vi "Subvi_Online_For_Offline_SWLDA_통합버전.vi"(0 "rate":dbl=500.0 caption="Rate" format="%0.2f", 1 "samples per channel":i32=25, 5 "Brain_data_source":dbl[][](array[numeric]) caption="EEG_Raw_Data" format="%0.3f", 7 "Target_Flash_Order":i64[][](array[numeric]), 8 "Value":T1, 9 "사용할 Parameter 갯수":i32=2, 10 "Weight":dbl[](array[numeric]), 11 "Path":path, 14 "Number":string, 16 "Matrix":T1, 17 "Channel selection":bool[](array[boolean])) -> (13 "LDA_Parameter":dbl[][](array[numeric]), 15 "EPR_발생_total":i16[](array[numeric]), 20 "output-0~8":i32, 22 "ERP_Parameters":dbl[][](array[numeric]))   [LabVIEW 2014]
uses:
  <vilib>/Analysis/Matrix/Datatypes/RealMatrix.ctl
  <vilib>/Analysis/3filter.llb/Filter Passband Type.ctl
  <vilib>/Analysis/baseanly.llb/Real A x B.vi
  <vilib>/Analysis/baseanly.llb/Mean (DBL).vi
  <vilib>/Analysis/3filter.llb/Butterworth Filter (DBL).vi
  <vilib>/Analysis/Matrix/Numeric/Conversions/Array To Matrix - RA.vi
  <vilib>/Analysis/Matrix/Numeric/Conversions/Array To Matrix - RA2.vi
  <vilib>/Analysis/Matrix/Numeric/Conversions/Matrix To Array - RM.vi
  <vilib>/Analysis/Matrix/Numeric/Multiply/Multiply - RM,RM.vi
  <vilib>/Analysis/Matrix/Numeric/Subtract/Subtract - RM,RM.vi
  <vilib>/Analysis/NI_AALBase.lvlib
  <vilib>/Analysis/Matrix/NI_Matrix.lvlib
  <vilib>/Utility/file.llb/Read From Spreadsheet File (DBL).vi
panel:
  out "Array 3":dbl[][](array[numeric])
  out "size(s)":i32[](array[numeric])
  out "A - B":T1
  out "Array 2":dbl[][](array[numeric])
  out "subarray":dbl[](array[numeric])
  out "Array":dbl[][](array[numeric])
  out "deleted portion":dbl[][](array[numeric])
  in  "LDA":path=path "C:/Users/Administrator/Desktop/공공복지안전사업연구-노수진/파일럿20130902/LDA_Matrix_Value.xls"
  out "#channel":i32
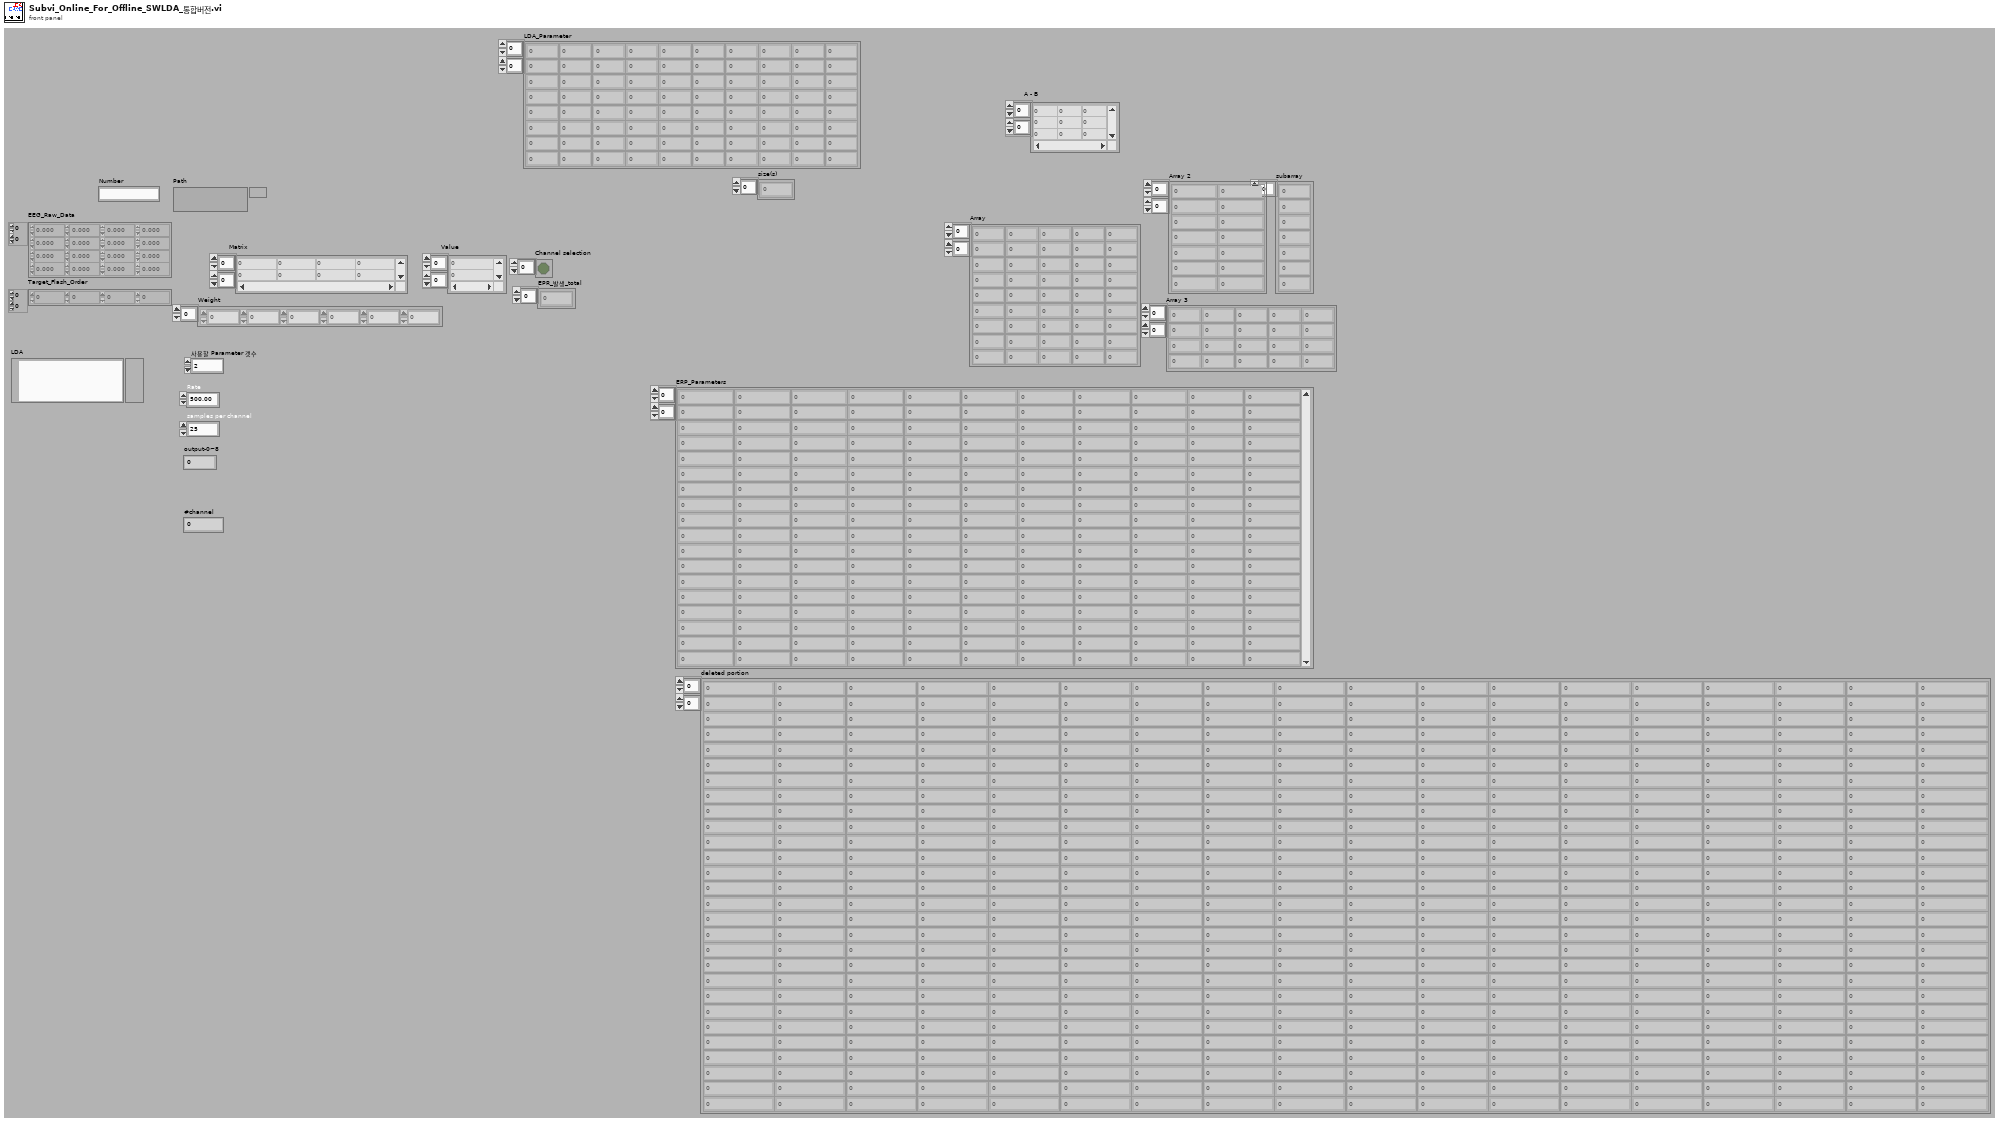
[diagram p1: front panel]
types:
  T1 = typedef "NI_Matrix.lvlib/RealMatrix.ctl" = dbl[][]
  T2 = typedef "NI_AALBase.lvlib/Filter Passband Type.ctl" = enum32{"Lowpass", "Highpass", "Bandpass", "Bandstop"}
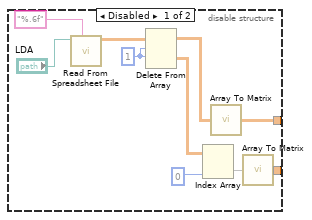
[diagram p3: hidden frame]
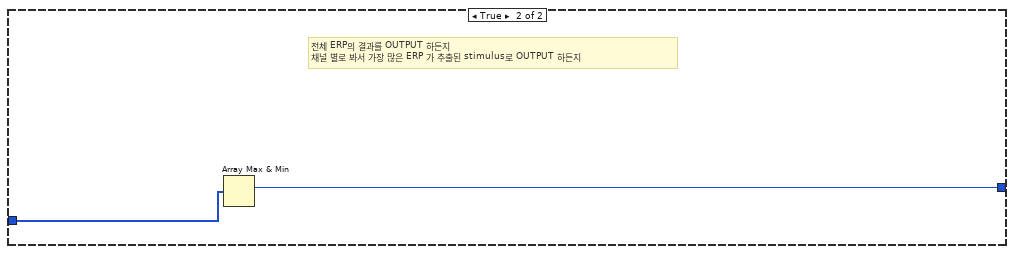
[diagram p4: hidden frame]
diagram:
  n1 = flat-sequence {
    tunnel: [w24] -> w19
    tunnel: [w48] -> w18
    tunnel: ["Target_Flash_Order"] -> w17
    tunnel: w19 -> [w48]
    tunnel: [w45] -> w16
    tunnel: w18 -> [w56]
    tunnel: w17 -> [w55]
    tunnel: w16 -> [w54]
    tunnel: [w52] -> w15
    tunnel: ["Weight"] -> w8
    tunnel: w15 -> [w183]
    tunnel: [w185] -> w14
    tunnel: [w185] -> w13
    tunnel: [w185] -> w12
    tunnel: w8 -> [w180]
    tunnel: [w180] -> w7
    tunnel: [w178] -> w5
    tunnel: w14 -> [_]
    tunnel: w13 -> [_]
    tunnel: w12 -> [w216]
    tunnel: [w219] -> w11
    tunnel: w7 -> [w218]
    tunnel: [w218] -> w6
    tunnel: w5 -> [w217]
    tunnel: [w216] -> w4
    tunnel: [w214] -> w2
    tunnel: w11 -> [w224]
    tunnel: [w224] -> w10
    tunnel: w6 -> [_]
    tunnel: w4 -> [w223]
    tunnel: [w223] -> w3
    tunnel: w2 -> [w222]
    tunnel: [w222] -> w1
    tunnel: [w227] -> w9
    tunnel: w10 -> [w228]
    tunnel: w3 -> [w226]
    tunnel: w1 -> [w225]
    tunnel: w9 -> [w233]
    frame #0 {
      n2 = Array Size(array="Brain_data_source") -> (size(s)=w25:i32[])
      n3 = Index Array(array=w25, index=1) -> (element=w27:i32)
      "#channel" <- w27
      n4 = for {
        N: w27 -> [_]
        tunnel: "Brain_data_source" -> [w32]
        shift-right: [w29] -> w21
        shift-left: dbl[][] [] ("Filtered X") -> [w30]
        tunnel: "Channel selection" -> [w28] mode=indexing
        i -> [w31]
        n5 = case shown="True" w28 {
          tunnel: w32 -> [_ w43]
          tunnel: w31 -> [_ w42]
          tunnel: w30 -> [w33 w36]
          tunnel: [w33 w35] -> w29
          frame False {
          }
          frame True {
            n6 = local read "rate"() -> (w37:dbl)
            n7 = Index Array(array=w43, index (col)=w42) -> (element=w41:dbl[])  [unwired: 1 in]
            n8 = call-poly <vilib>:"Butterworth Filter.vi"("filter type"=Filter_Passband_Type."Bandpass", "low cutoff freq: fl"=0.5, "high cutoff freq: fh"=30.0, "sampling freq: fs"=w37, "X"=w41) -> ("Filtered X"=w34:dbl[])  [unwired: 3 in, 1 out]
            n9 = Build Array (concatenate)(w36, w34) -> (w35:dbl[][])
          }
        }
      }
      n10 = Transpose 2D Array(2D array=w21) -> (transposed array=w24:dbl[][])
    }
    frame #1 {
      # "Bandpass per channel"
      # "20*9"
      n11 = Array Size(array="Target_Flash_Order") -> (size(s)=w47:i32[])
      n12 = Index Array(array=w47, index=1 ("인덱스")) -> (element=w45:i32)
    }
    frame #2 {
      (unwired) dbl[][] []
      (unwired) dbl[][] []
      n13 = for {
        N: w54 -> [_]
        tunnel: w56 -> [w69]
        tunnel: w55 -> [w68]
        shift-right: [w66] -> w52
        shift-left: dbl[][] [] -> [w65]
        shift-right: [w60] -> w50
        shift-left: dbl[][] [] -> [w59]
        tunnel: "Weight" -> [w58]
        i -> [w64]
        n14 = Index Array(array=w68, index (col)=w64) -> (element=w67:i64[])  [unwired: 1 in]
        n15 = flat-sequence {
          tunnel: w69 -> [w75]
          tunnel: w67 -> [w74]
          tunnel: [w73] -> w70
          tunnel: ["Path"] -> w63
          tunnel: ["Number"] -> w62
          tunnel: w70 -> [w136]
          tunnel: [w123] -> w57
          tunnel: w63 -> [_]
          tunnel: w62 -> [_]
          tunnel: [w118] -> w61
          tunnel: w58 -> [w126]
          frame #0 {
            # "10*600"
            # "Channel number"
            n16 = local read "samples per channel"() -> (w82:i32)
            n17 = local read "samples per channel"() -> (w81:i32)
            n18 = local read "rate"() -> (w84:dbl)
            n19 = Array Size(array=w75) -> (size(s)=w78:i32[])
            n20 = local read "rate"() -> (w86:dbl)
            n21 = Multiply(x=w84, y=0.2) -> (x*y=w88:dbl)
            n22 = Index Array(array=w78, index=1) -> (element=w80:i32)
            n23 = Add(x=w86, y=w88) -> (x+y=w87:dbl)
            n24 = Divide(x=w88, y=w82) -> (x/y=w85:dbl)
            n25 = Array Size(array=w74) -> (size(s)=w77:i32)
            n26 = for {
              N: w80 -> [_]
              tunnel: w81 -> [w89]
              tunnel: w87 -> [w100]
              shift-right: [w93] -> w73
              shift-left: dbl[][] [] -> [w95]
              tunnel: w77 -> [w94]
              tunnel: w75 -> [w92]
              tunnel: w74 -> [w91]
              tunnel: w85 -> [w90]
              i -> [w102]
              # "-20% ~ 100%: 1.2s epoch => 600 sample\ndim = 10*600 (ch# x 600 samp)"
              n27 = Initialize Array(0.0 ("element"), w100) -> (w99:dbl[])
              n28 = Index Array(array=w92, index (col)=w102) -> (element=w101:dbl[])  [unwired: 1 in]
              n29 = for {
                N: w94 -> [_]
                tunnel: w101 -> [w114]
                shift-right: [w111] -> w97
                shift-left: w99 -> [w112]
                tunnel: w100 -> [w110]
                tunnel: w91 -> [w108]
                tunnel: w90 -> [w106]
                tunnel: w89 -> [w104]
                i -> [w109]
                # "Average over each\nstimulus"
                # "20"
                n30 = Index Array(array=w108, index=w109) -> (element=w107:i64)
                n31 = Subtract(x=w107, y=w106) -> (x-y=w105:dbl)
                n32 = Multiply(x=w105, y=w104) -> (x*y=w103:dbl)
                n33 = Array Subset(array=w114, index=w103, length=w110) -> (w113:dbl[])
                n34 = Add(x=w113, y=w112) -> (x+y=w111:dbl[])
              }
              n35 = Divide(x=w97, y=w94) -> (x/y=w96:dbl[])
              n36 = Build Array (concatenate)(w95, w96) -> (w93:dbl[][])
            }
          }
          frame #1 {
            # "Weighted_Sum"
            # "epoch_size=600"
            # "250~450ms : P3 발생\n0~200 : N1 발생"
            # "10 + 1"
            n37 = Transpose 2D Array(2D array=w136) -> (transposed array=w124:dbl[][])
            n38 = Array Size(array=w124) -> (size(s)=w137:i32[])
            n39 = call-poly <vilib>:"Array To Matrix.vi"("Real 1D Array"=w126) -> ("Real Matrix (Column Vector)"=w132:T1)
            n40 = call-poly <vilib>:"Array To Matrix.vi"("Real 2D Array"=w124) -> ("Real Matrix"=w133:T1)
            n41 = Array Size(array=w124) -> (size(s)=w128:i32[])
            n42 = Index Array(array=w137, index #1=1 ("index"), index #2=0 ("인덱스")) -> (element #1=w134:i32)  [unwired: 1 out]
            n43 = Index Array(array=w128, index=0) -> (element=w127:i32)
            n44 = call-poly <vilib>:"A x B.vi"("B"=w132, "A"=w133) -> ("A x B"=w131:T1)  [unwired: 1 out]
            n45 = call-poly <vilib>:"Matrix To Array.vi"("Real Matrix"=w131) -> ("Real 2D Array"=w129:dbl[][])
            n46 = Increment(x=w134) -> (x+1=w122:i32)
            n47 = Reshape Array(w129, w127) -> (w125:dbl[])
            n48 = Insert Into Array(array=w124, index (col)=w134, new element=w125) -> (w121:dbl[][])  [unwired: 1 in]
            n49 = for {
              N: w122 -> [_]
              tunnel: w121 -> [w168]
              tunnel: [w146] -> _ mode=indexing
              tunnel: [w145] -> _ mode=indexing
              tunnel: [w144] -> _ mode=indexing
              tunnel: [w143] -> _ mode=indexing
              tunnel: [w142] -> w120 mode=indexing
              shift-right: [w139] -> w118
              shift-left: dbl[][] [] -> [w141]
              i -> [w153]
              n50 = local read "rate"() -> (w167:dbl)
              n51 = Index Array(array=w168, index (col)=w153) -> (element=w158:dbl[])  [unwired: 1 in]
              n52 = Multiply(x=w167, y=0.2) -> (x*y=w165:dbl)
              n53 = Split 1D Array(array=w158, index=w165) -> (first subarray=w164:dbl[], second subarray=w149:dbl[])
              n54 = local read "rate"() -> (w161:dbl)
              n55 = call-poly <vilib>:"Mean.vi"("X"=w164) -> ("mean"=w163:dbl)  [unwired: 1 out]
              n56 = Multiply(x=w161, y=0.1) -> (x*y=w147:dbl)
              n57 = Subtract(x=w149, y=w163) -> (x-y=w140:dbl[])
              n58 = Divide(x=w161, y=w147) -> (x/y=w160:dbl)
              n59 = for {
                N: w160 -> [_]
                tunnel: w140 -> [w173]
                tunnel: [w174] -> w157 mode=indexing
                tunnel: w147 -> [w171]
                i -> [w170]
                n60 = Multiply(x=w170, y=w171) -> (x*y=w172:dbl)
                n61 = Array Subset(array=w173, index=w172, length=w171) -> (w169:dbl[])
                n62 = call-poly <vilib>:"Mean.vi"("X"=w169) -> ("mean"=w174:dbl)  [unwired: 1 out]
              }
              n63 = Build Array (concatenate)(w141, w140) -> (w139:dbl[][])
              n64 = Array Max & Min(array=w157) -> (max index (indices)=w152:i32)  [unwired: 3 out]
              n65 = Array Max & Min(array=w157) -> (min index (indices)=w151:i32)  [unwired: 3 out]
              n66 = Multiply(x=w152, y=w147) -> (x*y=w148:dbl)
              n67 = Multiply(x=w151, y=w147) -> (x*y=w155:dbl)
              n68 = Array Subset(array=w140, index=w148, length=w147) -> (w150:dbl[])
              n69 = Array Subset(array=w140, index=w155, length=w147) -> (w156:dbl[])
              n70 = Array Max & Min(array=w156) -> (min value=w144:dbl, min index (indices)=w154:i32)  [unwired: 2 out]
              n71 = Array Max & Min(array=w150) -> (max value=w146:dbl, max index (indices)=w159:i32)  [unwired: 2 out]
              n72 = Add(x=w159, y=w148) -> (x+y=w145:dbl)
              n73 = Add(x=w155, y=w154) -> (x+y=w143:dbl)
              n74 = Build Array(w146, w145, w144, w143) -> (w142:dbl[])
            }
            "Array 3" <- w120
            n75 = global read "Control_Panel.vi" "EEG_Channel_Num"() -> (w115:i32)
            n76 = call "Reshape2.vi"("Numeric"=4, "EEG_Channel_Num"=w115, "all rows"=w120, "Numeric 2"=1.0) -> ("Array"=w123:dbl[][])  [unwired: 7 in]
          }
        }
        n77 = Build Array (concatenate)(w59, w61) -> (w60:dbl[][])
        n78 = Build Array (concatenate)(w65, w57) -> (w66:dbl[][])
        "Array" <- w57
      }
      "ERP_Parameters" <- w52
      "LDA_Parameter" <- w50
    }
    frame #3 {
      # "여기 틀림"
      # "ERP_Parameter\n\n1. P3_Amp\n2. P3_Latency\n3. N1_Amp\n4. N1_Latency"
      n79 = disable-structure shown="Enabled" {
        disable-tunnel: [w192 "Matrix"] -> w177
        disable-tunnel: [w191 "Value"] -> w184
        frame Disabled {
          w194 = 1 ("인덱스 (행)")
          n80 = call-poly <vilib>:"Read From Spreadsheet File.vi"("format (%.3f)"="%.6f", "file path (dialog if empty)"="LDA") -> ("all rows"=w188:dbl[][])  [unwired: 5 in, 4 out]
          n81 = Delete From Array(array=w188, length=w194, index (row)=w194) -> (deleted portion=w197:dbl[][], array with subset deleted=w196:dbl[][])  [unwired: 1 in]
          n82 = Index Array(array=w197, index (col)=0 ("인덱스")) -> (element=w195:dbl[])  [unwired: 1 in]
          n83 = call-poly <vilib>:"Array To Matrix.vi"("Real 2D Array"=w196) -> ("Real Matrix"=w192:T1)
          n84 = call-poly <vilib>:"Array To Matrix.vi"("Real 1D Array"=w195) -> ("Real Matrix (Column Vector)"=w191:T1)
        }
        frame Enabled {
        }
      }
      n85 = Delete From Array(array=w183, length="사용할 Parameter 갯수", index (col)=0 ("비활성화된 인덱스 (열)")) -> (deleted portion=w182:dbl[][])  [unwired: 1 in, 1 out]
      "deleted portion" <- w182
      n86 = for {
        tunnel: w177 -> [w204]
        tunnel: w184 -> [w211]
        shift-right: [w209] -> w186
        shift-left: dbl[][] [] -> [w208]
        tunnel: w182 -> [w207] mode=indexing
        n87 = call-poly <vilib>:"Array To Matrix.vi"("Real 1D Array"=w207) -> ("Real Matrix (Column Vector)"=w205:T1)
        n88 = call-poly <vilib>:"Multiply.vi"("Real Matrix B"=w205, "Real Matrix A"=w204) -> ("A * B"=w206:T1)
        "A - B" <- w206
        n89 = call-poly <vilib>:"Subtract.vi"("Real Matrix B"=w211, "Real Matrix A"=w206) -> ("A - B"=w212:T1)
        n90 = call-poly <vilib>:"Matrix To Array.vi"("Real Matrix"=w212) -> ("Real 2D Array"=w210:dbl[][])
        n91 = Build Array (concatenate)(w208, w210) -> (w209:dbl[][])
      }
      "Array 2" <- w186
      n92 = Array Size(array=w177) -> (size(s)=→"size(s)":i32[])
      n93 = Index Array(array=w186, index (col)=0 ("비활성화된 인덱스 (열)")) -> (element=w178:dbl[])  [unwired: 1 in]
      "subarray" <- w178
      n94 = for {
        tunnel: w178 -> [w203] mode=indexing
        tunnel: [w202] -> w185 mode=indexing
        n95 = Greater?(x=w203, y=0.0) -> (0:w200:bool)
        n96 = Boolean To (0,1)(Boolean=w200) -> (0, 1=w202:i16)
      }
    }
    frame #4 {
      n97 = Multiply(x=w216, y=w217) -> (x*y=w215:dbl[])
      n98 = Multiply(x=w215, y=-1) -> (x*y=w214:dbl[])
      n99 = Add Array Elements(numeric array=w216) -> (sum=w221:i16)
      n100 = Equal?(x=w221, y=i16 1) -> (x = y?=w219:bool)
      "EPR_발생_total" <- w216
    }
    frame #5 {
      # "#1> #2\n참에서는 참으로만\n참에서 거짓: 불가능\n거짓에서 참: 가능 (전체에선 단독 ERP가 안나왔지만 채널 별로 보니까 나옴)"
      # "#1"
    }
    frame #6 {
      # "#2"
      n101 = case shown="False" w228 {
        tunnel: [w230 w232] -> w227
        tunnel: w226 -> [_ w231]
        tunnel: w225 -> [w229 _]
        frame False {
          n102 = Array Max & Min(array=w229) -> (max index (indices)=w230:i32)  [unwired: 3 out]
        }
        frame True {
          # "전체 ERP의 결과를 OUTPUT 하든지\n채널 별로 봐서 가장 많은 ERP 가 추출된 stimulus로 OUTPUT 하든지"
          n103 = Array Max & Min(array=w231) -> (max index (indices)=w232:i32)  [unwired: 3 out]
        }
      }
    }
    frame #7 {
      "output-0~8" <- w233
    }
  }
